vi "Wolna_sprawdz_buf_size.vi"(6 "Okres in":dbl, 8 "error in (no error)":errorcluster, 9 "Data in":T1) -> (0 "error out":errorcluster, 1 "Data out":T1, 2 "bufor OK?":bool, 3 "Okres out":dbl)   [LabVIEW 2013]
doc: "Sprawdza czy rozmiar bufora danych jest wiêkszy lub równy\nliczbie próbek równej okresowi jednego pomiaru"
uses:
  Kontrolki/Przetwarzanie/Kanaly.ctl
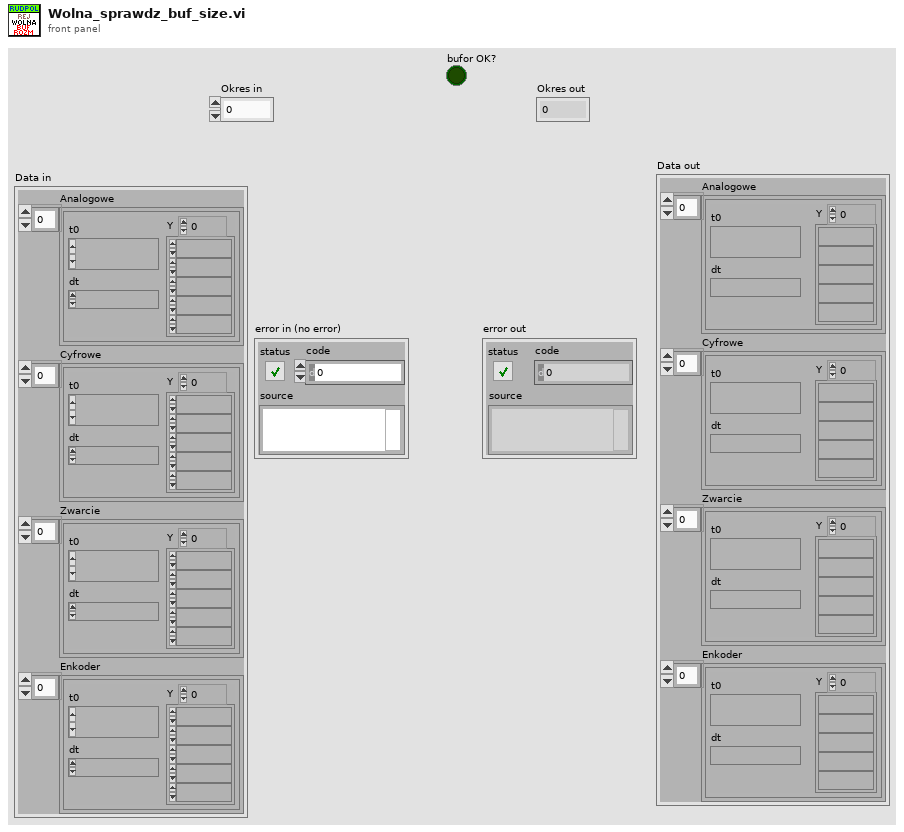
[diagram p1: front panel]
types:
  T1 = typedef "Kanaly.ctl" = cluster{"Analogowe":waveform(dbl)[], "Cyfrowe":waveform(dbl)[], "Zwarcie":waveform(dbl)[], "Enkoder":waveform(dbl)[]}
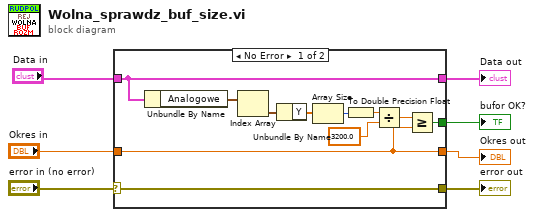
[diagram p0: block diagram]
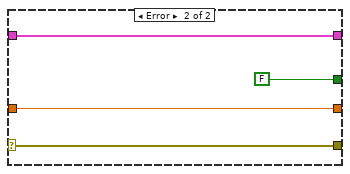
[diagram p2: hidden frame]
diagram:
  n1 = case shown="No Error" "error in (no error)" {
    selector: "error in (no error)" -> [w12 w21]
    tunnel: "Okres in" -> [w10 w19]
    tunnel: [w8 w22] -> w1
    tunnel: "Data in" -> [w8 w22]
    tunnel: [w12 w21] -> w5
    tunnel: [w11 FALSE] -> w4
    tunnel: [w10 w19] -> w3
    frame No Error {
      n2 = Unbundle By Name(w8) -> ("Analogowe"=w9:waveform(dbl)[])
      n3 = Index Array(array=w9) -> (element=w18:waveform(dbl))  [unwired: 1 in]
      n4 = Unbundle By Name(w18) -> ("Y"=w17:dbl[])
      n5 = Array Size(array=w17) -> (size(s)=w15:i32)
      n6 = To Double Precision Float(number=w15) -> (double precision float=w14:dbl)
      n7 = Divide(x=w14, y=3200.0) -> (x/y=w16:dbl)
      n8 = Greater Or Equal?(x=w16, y=w10) -> (x >= y?=w11:bool)
    }
    frame Error {
    }
  }
  "error out" <- w5
  "bufor OK?" <- w4
  "Okres out" <- w3
  "Data out" <- w1
